vi "Tausand AB1000 Delay Sweep Example (StateMachine).vi"() -> ()   [LabVIEW 2015]
doc: "Example of a delay sweep with a Tausand Abacus AB1002 or AB1004 device.\n\nVerifies if the selected port is valid, then changes the delay in the given range. Measures a single time at each delay. Produces live graphics.\nUses only inputs in channels A and B.\nBlock diagram coded as a state machine."
uses:
  <instrlib>/Tausand AB1000/Public/Controls/counters2ch.ctl
  <instrlib>/Tausand AB1000/Examples/sub vi/delaySweep_states.ctl
  <instrlib>/Tausand AB1000/Public/Controls/deviceTypeRing.ctl
  <instrlib>/Tausand AB1000/Public/Controls/channelRing.ctl
  <instrlib>/Tausand AB1000/Tausand AB1000.lvlib
panel:
  out "counters":T1
  out "device type":T2 items=["any"=0, "AB1002"=1002, "AB1004"=1004]
  in  "step":i32=5 min=5 max=100 step=5
  out "progressStr":string
  out "current delay":i32
  out "valid data?":bool
  out "dataID":u32
  out "Total progress":dbl(slide) scale=0.0..100.0
  out "number of delays":i32
  out "delay index":i32
  out "state":T3
  out "counters array":T1[](array[typedef])
  out "wait done?":bool
  out "nextRead":u32 caption="next read in (s)"
  out "current time":timestamp
  out "wait until":timestamp
  in  "stop":bool
  out "delay array":i32[](array[numeric])
  out "BGrph":cluster{i32[], u32[]}(graph)
  out "AGrph":cluster{i32[], u32[]}(graph)
  out "coincGrph":cluster{i32[], u32[]}(graph)
  out "Delay A (ns)":u32
  out "Delay B (ns)":u32=5
  in  "Delay range (ns)":cluster{i32, i32}(slide)={-20, 20} scale=-100.0..100.0
  in  "Device settings":T4={"Sampling time (ms)"=1000, "Coincidence window (ns)"=5, "Delay A (ns)"=0, "Delay B (ns)"=0, "Sleep time A (ns)"=0, "Sleep time B (ns)"=0} {"Sleep time B (ns)" max=100 step=5; "Sleep time A (ns)" max=100 step=5; "Coincidence window (ns)" max=50000 step=5; "Sampling time (ms)" items=["1000s"=1000000, "500s"=500000, "200s"=200000, "100s"=100000, "50s"=50000, "20s"=20000, "10s"=10000, "5s"=5000, "2s"=2000, "1s"=1000, "500ms"=500, "200ms"=200, "100ms"=100, "50ms"=50, "20ms"=20, "10ms"=10, "5ms"=5, "2ms"=2, "1ms"=1]}
  out "valid device?":bool
  in  "VISA port":refnum<visa-resource-name>
  # "Overview: example doing a delay sweep in a Tausand Abacus AB1002 or AB1004 device.\nInstructions:\n1. Select the VISA port.\n2. Enter the desired settings.\n3. Run the VI.\n4. Click stop to abort the VI execution."
  # "April 2019"
  # "Set these values before running the VI."
  # "Counts at last delay:"
  # "Delay in progess:"
  # "ns"
  # "Positive delay:   A delayed,        B not delayed\nNegative delay: A not delayed, B delayed"
  # "from"
  # "to"
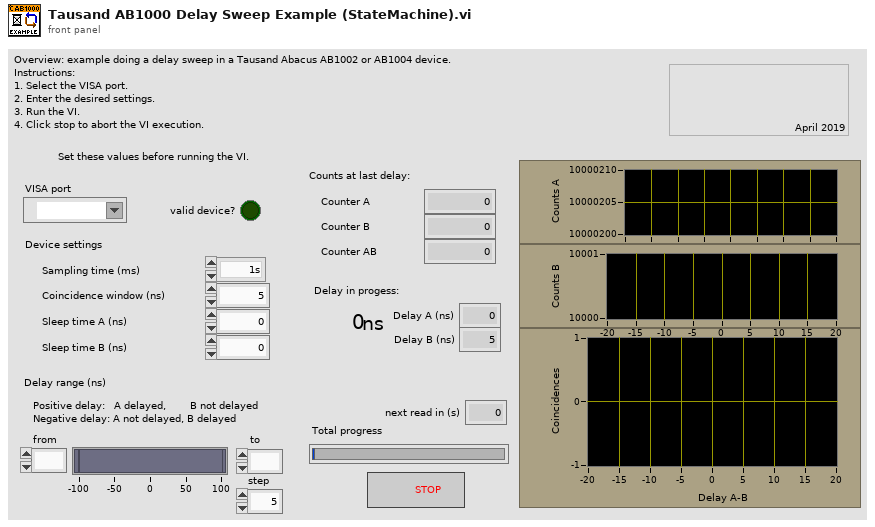
[diagram p1: front panel]
types:
  T1 = typedef "Tausand AB1000.lvlib/counters2ch.ctl" = cluster{"counter_A":u32, "counter_B":u32, "counter_AB":u32, "counters_ID":u32, "time_left":u32}
  T2 = typedef "Tausand AB1000.lvlib/deviceTypeRing.ctl" = u16
  T3 = typedef "delaySweep_states.ctl" = enum16{"update delay range", "create delay array", "verify port", "invalid port message", "create counter array", "initialize device", "set delay", "set wait timer", "wait sampling time", "read data", "graph data", "increase index", "repeat measurement", "close device", "end state"}
  T4 = cluster{"Sampling time (ms)":u32, "Coincidence window (ns)":u32, "Delay A (ns)":u32, "Delay B (ns)":u32, "Sleep time A (ns)":u32, "Sleep time B (ns)":u32}
  T5 = typedef "Tausand AB1000.lvlib/channelRing.ctl" = u8
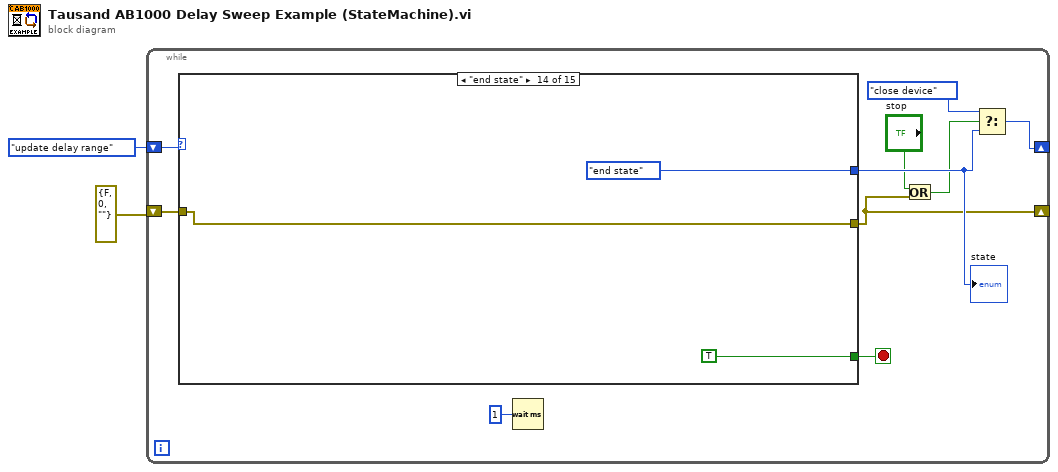
[diagram p0: block diagram]
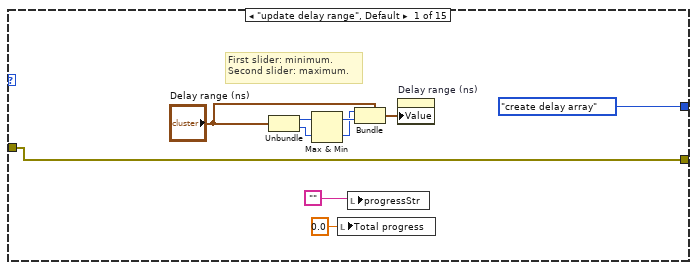
[diagram p2: hidden frame]
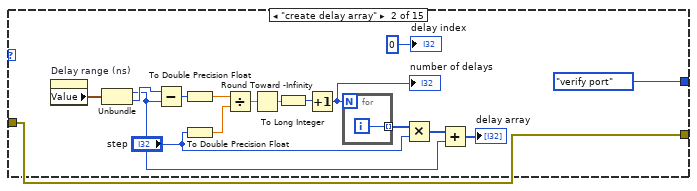
[diagram p3: hidden frame]
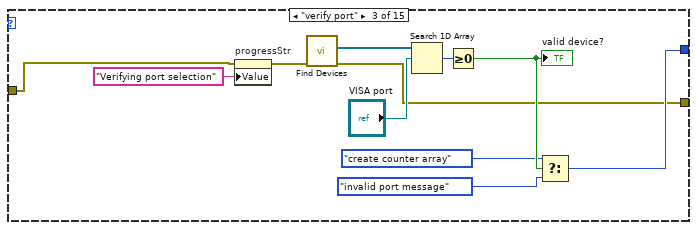
[diagram p4: hidden frame]
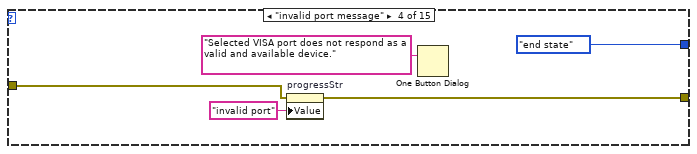
[diagram p5: hidden frame]
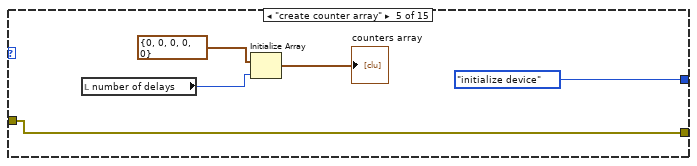
[diagram p6: hidden frame]
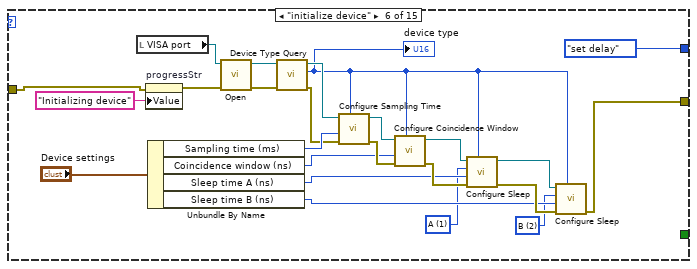
[diagram p7: hidden frame]
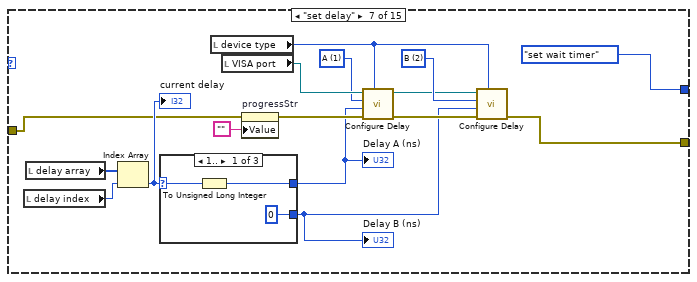
[diagram p8: hidden frame]
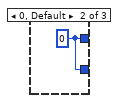
[diagram p9: hidden frame]
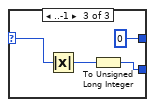
[diagram p10: hidden frame]
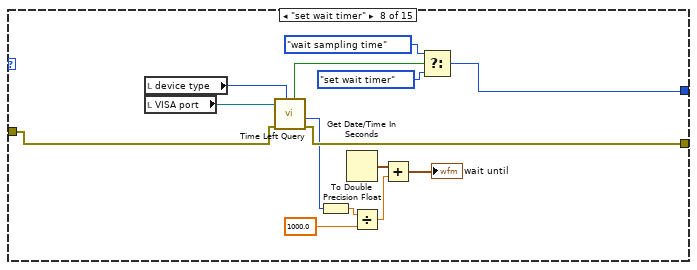
[diagram p11: hidden frame]
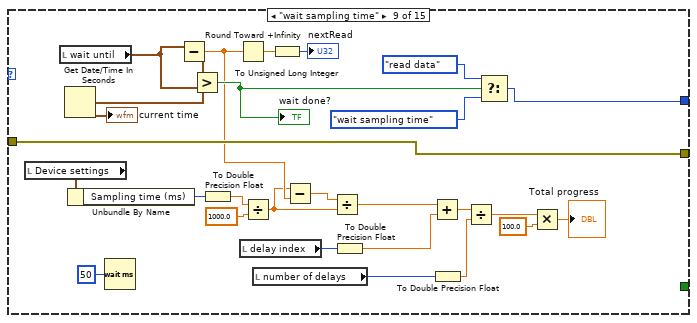
[diagram p12: hidden frame]
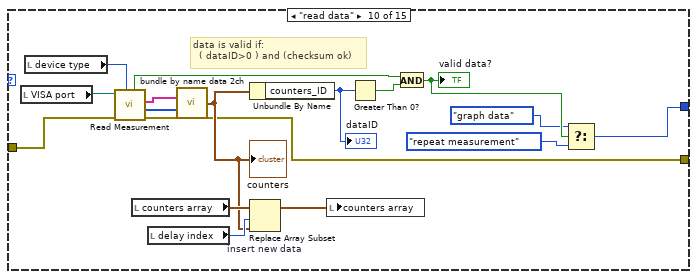
[diagram p13: hidden frame]
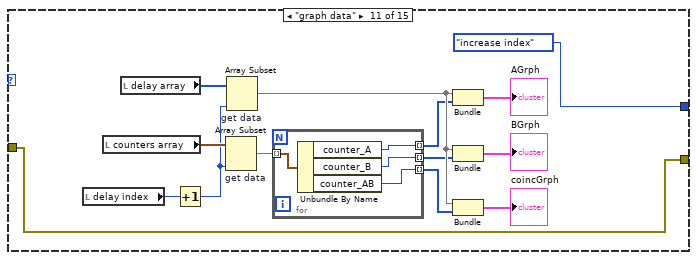
[diagram p14: hidden frame]
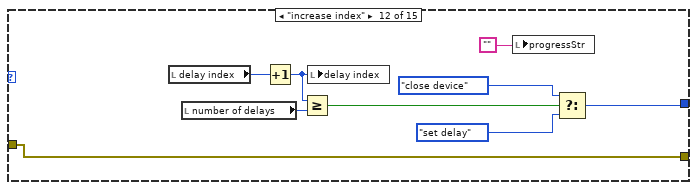
[diagram p15: hidden frame]
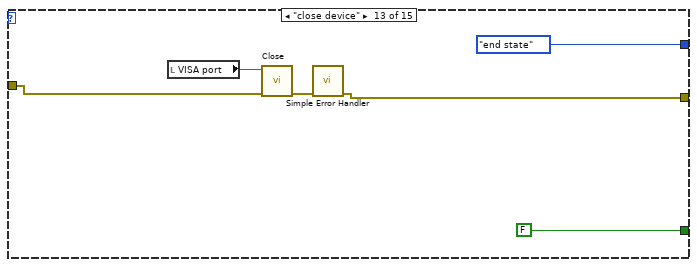
[diagram p16: hidden frame]
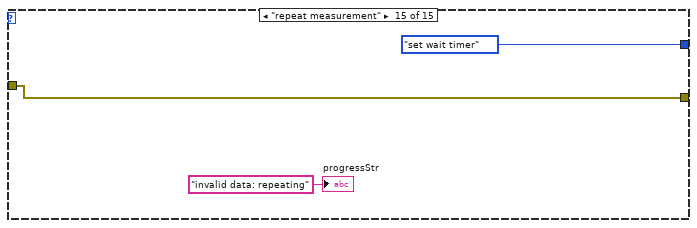
[diagram p17: hidden frame]
diagram:
  n1 = while {
    shift-right: [w6] -> _
    shift-left: delaySweep_states."update delay range" -> [w12]
    shift-right: [w5] -> _
    shift-left: errorcluster {"status"=FALSE, "code"=0, "source"=""} ("error in (no error)") -> [w10]
    stop <- w9 stop-if-true
    n2 = case shown="\"end state\"" w12 {
      tunnel: [delaySweep_states."create delay array" delaySweep_states."verify port" w46 delaySweep_states."end state" delaySweep_states."initialize device" delaySweep_states."set delay" delaySweep_states."set wait timer" w112 w141 w159 delaySweep_states."increase index" w186 delaySweep_states."end state" delaySweep_states."end state" delaySweep_states."set wait timer"] -> w7
      tunnel: [_ _ _ _ _ _ _ _ _ _ _ _ FALSE TRUE _] -> w9
      tunnel: w10 -> [w15 w28 w43 w53 w58 w82 w96 w117 w149 w156 w179 w193 w196 w200 w205]
      tunnel: [w15 w28 w41 w52 w58 w65 w87 w116 w149 w151 w179 w193 w195 w200 w205] -> w5
      frame "update delay range", Default {
        # "First slider: minimum.\nSecond slider: maximum."
        n3 = Unbundle("Delay range (ns)") -> (w22:i32, w17:i32)
        n4 = Max & Min(x=w22, y=w17) -> (max(x,y)=w19:i32, min(x,y)=w16:i32)
        n5 = local write "Total progress"(0.0 ("Total progress")) -> ()
        n6 = local write "progressStr"("") -> ()
        n7 = Bundle(cluster="Delay range (ns)", w16, w19) -> (w20:cluster{i32, i32})
        n8 = property on="Delay range (ns)" class="Slide (strict)"("Value"=w20) -> ()  [unwired: 2 in, 2 out]
      }
      frame "create delay array" {
        n9 = property on="Delay range (ns)" class="Slide (strict)"() -> ("Value"=w31:cluster{i32, i32})  [unwired: 2 in, 2 out]
        n10 = Unbundle(w31) -> (w29:i32, w30:i32)
        n11 = Subtract(x=w30, y=w29) -> (x-y=w38:i32)
        n12 = To Double Precision Float(number=w38) -> (double precision float=w36:dbl)
        n13 = To Double Precision Float(number="step") -> (double precision float=w35:dbl)
        n14 = Divide(x=w36, y=w35) -> (x/y=w24:dbl)
        n15 = Round Toward -Infinity(1:w24) -> (0:w23:dbl)
        n16 = To Long Integer(number=w23) -> (32bit integer=w32:i32)
        n17 = Increment(x=w32) -> (x+1=w25:i32)
        "number of delays" <- w25
        n18 = for {
          N: w25 -> [_]
          tunnel: [w40] -> w37 mode=indexing
          i -> [w40]
        }
        n19 = Multiply(x=w37, y="step") -> (x*y=w33:i32[])
        n20 = Add(x=w33, y=w29) -> (x+y=→"delay array":i32[])
        "delay index" <- 0 ("delay index")
      }
      frame "verify port" {
        n21 = property on="progressStr" class="Str"(error in=w43, "Value"="Verifying port selection" ("progressStr")) -> (error out=w42:errorcluster)  [unwired: 1 in, 1 out]
        n22 = call <instrlib>:"Find Devices.vi"("error in (no error)"=w42) -> ("error out"=w41:errorcluster, "Abacus VISAs"=w49:refnum<visa-resource-name>[])  [unwired: 8 in, 1 out]
        n23 = Search 1D Array(1D array=w49, element="VISA port") -> (index of element=w51:i32)  [unwired: 1 in]
        n24 = Greater Or Equal To 0?(x=w51) -> (x >= 0?=w48:bool)
        "valid device?" <- w48
        n25 = Select(t=delaySweep_states."create counter array", s=w48, f=delaySweep_states."invalid port message") -> (s? t:f=w46:T3)
      }
      frame "invalid port message" {
        n26 = property on="progressStr" class="Str"(error in=w53, "Value"="invalid port" ("progressStr")) -> (error out=w52:errorcluster)  [unwired: 1 in, 1 out]
        n27 = One Button Dialog(message="Selected VISA port does not respond as a valid and available device.") -> ()  [unwired: 1 in, 1 out]
      }
      frame "create counter array" {
        n28 = local read "number of delays"() -> (w57:i32)
        n29 = Initialize Array "Initialize Array"(T1 {"counter_A"=0, "counter_B"=0, "counter_AB"=0, "counters_ID"=0, "time_left"=0} ("counters"), w57) -> (→"counters array":T1[])
      }
      frame "initialize device" {
        w67 = T5 2 items=["none", "A", "B", "C", "D", "E", "F", "G", "H"] ("channel")
        w68 = T5 1 items=["none", "A", "B", "C", "D", "E", "F", "G", "H"] ("channel")
        n30 = local read "VISA port"() -> (w84:refnum<visa-resource-name>)
        n31 = property on="progressStr" class="Str"(error in=w82, "Value"="Initializing device" ("progressStr")) -> (error out=w81:errorcluster)  [unwired: 1 in, 1 out]
        n32 = Unbundle By Name("Device settings") -> ("Sampling time (ms)"=w72:u32, "Coincidence window (ns)"=w71:u32, "Sleep time A (ns)"=w70:u32, "Sleep time B (ns)"=w69:u32)
        n33 = call <instrlib>:"Open.vi"("error in (no error)"=w81, "VISA resource name"=w84) -> ("error out"=w79:errorcluster, "VISA resource name out"=w80:refnum<visa-resource-name>)  [unwired: 8 in]
        n34 = call <instrlib>:"Device Type Query.vi"("error in (no error)"=w79, "VISA Refnum in"=w80) -> ("error out"=w66:errorcluster, "device type"=w62:T2, "VISA Refnum out"=w64:refnum<visa-resource-name>)  [unwired: 7 in]
        "device type" <- w62
        n35 = call <instrlib>:"Configure Sampling Time.vi"("device type"=w62, "error in (no error)"=w66, "value (1000 ms)"=w72, "VISA Refnum in"=w64) -> ("error out"=w78:errorcluster, "VISA Refnum out"=w77:refnum<visa-resource-name>)  [unwired: 5 in, 1 out]
        n36 = call <instrlib>:"Configure Coincidence Window.vi"("device type"=w62, "error in (no error)"=w78, "value ns (10ns)"=w71, "VISA Refnum in"=w77) -> ("error out"=w75:errorcluster, "VISA Refnum out"=w76:refnum<visa-resource-name>)  [unwired: 5 in, 1 out]
        n37 = call <instrlib>:"Configure Sleep.vi"("device type"=w62, "error in (no error)"=w75, "value (0 ns)"=w70, "channel"=w68, "VISA Refnum in"=w76) -> ("error out"=w73:errorcluster, "VISA Refnum out"=w74:refnum<visa-resource-name>)  [unwired: 4 in, 1 out]
        n38 = call <instrlib>:"Configure Sleep.vi"("device type"=w62, "error in (no error)"=w73, "value (0 ns)"=w69, "channel"=w67, "VISA Refnum in"=w74) -> ("error out"=w65:errorcluster)  [unwired: 4 in, 2 out]
      }
      frame "set delay" {
        w90 = T5 2 items=["none", "A", "B", "C", "D", "E", "F", "G", "H"] ("channel")
        w91 = T5 1 items=["none", "A", "B", "C", "D", "E", "F", "G", "H"] ("channel")
        n39 = local read "delay index"() -> (w98:i32)
        n40 = local read "delay array"() -> (w100:i32[])
        n41 = Index Array(array=w100, index=w98) -> (element=w99:i32)
        "current delay" <- w99
        n42 = case shown="1.." w99 {
          selector: w99 -> [w102 _ w107]
          tunnel: [u32 0 w105 w109] -> w89
          tunnel: [w104 w105 u32 0 ("Delay A (ns)")] -> w92
          frame 1.. {
            n43 = To Unsigned Long Integer(number=w102) -> (unsigned 32bit integer=w104:u32)
          }
          frame 0, Default {
            w105 = u32 0 ("Delay A (ns)")
          }
          frame ..-1 {
            n44 = Absolute Value(x=w107) -> (abs(x)=w106:i32)
            n45 = To Unsigned Long Integer(number=w106) -> (unsigned 32bit integer=w109:u32)
          }
        }
        "Delay A (ns)" <- w92
        "Delay B (ns)" <- w89
        n46 = local read "device type"() -> (w86:T2)
        n47 = local read "VISA port"() -> (w95:refnum<visa-resource-name>)
        n48 = property on="progressStr" class="Str"(error in=w96, "Value"="" ("progressStr")) -> (error out=w93:errorcluster)  [unwired: 1 in, 1 out]
        n49 = call <instrlib>:"Configure Delay.vi"("device type"=w86, "error in (no error)"=w93, "value (0 ns)"=w92, "channel"=w91, "VISA Refnum in"=w95) -> ("error out"=w94:errorcluster, "VISA Refnum out"=w88:refnum<visa-resource-name>)  [unwired: 4 in, 1 out]
        n50 = call <instrlib>:"Configure Delay.vi"("device type"=w86, "error in (no error)"=w94, "value (0 ns)"=w89, "channel"=w90, "VISA Refnum in"=w88) -> ("error out"=w87:errorcluster)  [unwired: 4 in, 2 out]
      }
      frame "set wait timer" {
        n51 = local read "device type"() -> (w110:T2)
        n52 = local read "VISA port"() -> (w118:refnum<visa-resource-name>)
        n53 = call <instrlib>:"Time Left Query.vi"("device type"=w110, "error in (no error)"=w117, "VISA Refnum in"=w118) -> ("error out"=w116:errorcluster, "time left ms out"=w115:u32, "checksum ok?"=w114:bool)  [unwired: 5 in, 1 out]
        n54 = To Double Precision Float(number=w115) -> (double precision float=w119:dbl)
        n55 = Get Date/Time In Seconds() -> (seconds since 1Jan1904=w122:timestamp)
        n56 = Divide(x=w119, y=1000.0) -> (x/y=w120:dbl)
        n57 = Add(x=w122, y=w120) -> (x+y=→"wait until":timestamp)
        n58 = Select(t=delaySweep_states."wait sampling time", s=w114, f=delaySweep_states."set wait timer") -> (s? t:f=w112:T3)
      }
      frame "wait sampling time" {
        n59 = local read "Device settings"() -> (w128:T4)
        n60 = local read "wait until"() -> (w147:timestamp)
        n61 = Get Date/Time In Seconds() -> (seconds since 1Jan1904=w148:timestamp)
        "current time" <- w148
        n62 = Unbundle By Name(w128) -> ("Sampling time (ms)"=w125:u32)
        n63 = Wait (ms)(milliseconds to wait=u32 50) -> ()  [unwired: 1 out]
        n64 = Subtract(x=w147, y=w148) -> (x-y=w136:dbl)
        n65 = Greater?(x=w148, y=w147) -> (0:w144:bool)
        "wait done?" <- w144
        n66 = To Double Precision Float(number=w125) -> (double precision float=w127:dbl)
        n67 = Round Toward +Infinity(x=w136) -> (ceil(x): smallest int >= x=w146:dbl)
        n68 = local read "delay index"() -> (w132:i32)
        n69 = Divide(x=w127, y=1000.0) -> (x/y=w124:dbl)
        n70 = local read "number of delays"() -> (w133:i32)
        n71 = To Unsigned Long Integer(number=w146) -> (unsigned 32bit integer=→"nextRead":u32)
        n72 = Subtract(x=w124, y=w136) -> (x-y=w135:dbl)
        n73 = Divide(x=w135, y=w124) -> (x/y=w134:dbl)
        n74 = To Double Precision Float(number=w132) -> (double precision float=w131:dbl)
        n75 = Add(x=w134, y=w131) -> (x+y=w137:dbl)
        n76 = To Double Precision Float(number=w133) -> (double precision float=w129:dbl)
        n77 = Divide(x=w137, y=w129) -> (x/y=w139:dbl)
        n78 = Select(t=delaySweep_states."read data", s=w144, f=delaySweep_states."wait sampling time") -> (s? t:f=w141:T3)
        n79 = Multiply(x=w139, y=100.0) -> (x*y=→"Total progress":dbl)
      }
      frame "read data" {
        # "data is valid if:\n  ( dataID>0 ) and (checksum ok)"
        n80 = local read "VISA port"() -> (w157:refnum<visa-resource-name>)
        n81 = local read "device type"() -> (w150:T2)
        n82 = call <instrlib>:"Read Measurement.vi"("device type"=w150, "error in (no error)"=w156, "VISA Refnum in"=w157) -> ("error out"=w151:errorcluster, "values"=w154:u32[], "labels"=w155:string[], "checksum ok?"=w152:bool)  [unwired: 3 in, 2 out]
        n83 = local read "counters array"() -> (w165:T1[])
        n84 = local read "delay index"() -> (w164:i32)
        n85 = call <instrlib>:"bundle by name data 2ch.vi"("names"=w155, "values"=w154) -> ("output cluster 2ch"=w153:T1)  [unwired: 13 in]
        "counters" <- w153
        n86 = Unbundle By Name(w153) -> ("counters_ID"=w158:u32)
        "dataID" <- w158
        n87 = Replace Array Subset "insert new data"(array=w165, new element=w153, index=w164) -> (w166:T1[])
        n88 = local write "counters array"(w166) -> ()
        n89 = Greater Than 0?(x=w158) -> (x > 0?=w163:bool)
        n90 = And(x=w152, y=w163) -> (x .and. y?=w162:bool)
        "valid data?" <- w162
        n91 = Select(t=delaySweep_states."graph data", s=w162, f=delaySweep_states."repeat measurement") -> (s? t:f=w159:T3)
      }
      frame "graph data" {
        n92 = local read "delay index"() -> (w168:i32)
        n93 = local read "counters array"() -> (w169:T1[])
        n94 = local read "delay array"() -> (w170:i32[])
        n95 = Increment(x=w168) -> (x+1=w167:i32)
        n96 = Array Subset "get data"(array=w169, length=w167) -> (w174:T1[])  [unwired: 1 in]
        n97 = Array Subset "get data"(array=w170, length=w167) -> (w175:i32[])  [unwired: 1 in]
        n98 = for {
          tunnel: w174 -> [w184] mode=indexing
          tunnel: [w183] -> w173 mode=indexing
          tunnel: [w182] -> w172 mode=indexing
          tunnel: [w181] -> w171 mode=indexing
          n99 = Unbundle By Name(w184) -> ("counter_A"=w183:u32, "counter_B"=w182:u32, "counter_AB"=w181:u32)
        }
        n100 = Bundle(w175, w173) -> (→"AGrph":cluster{i32[], u32[]})  [unwired: 1 in]
        n101 = Bundle(w175, w172) -> (→"BGrph":cluster{i32[], u32[]})  [unwired: 1 in]
        n102 = Bundle(w175, w171) -> (→"coincGrph":cluster{i32[], u32[]})  [unwired: 1 in]
      }
      frame "increase index" {
        n103 = local read "delay index"() -> (w192:i32)
        n104 = local read "number of delays"() -> (w190:i32)
        n105 = Increment(x=w192) -> (x+1=w191:i32)
        n106 = Greater Or Equal?(x=w191, y=w190) -> (x >= y?=w189:bool)
        n107 = local write "delay index"(w191) -> ()
        n108 = local write "progressStr"("") -> ()
        n109 = Select(t=delaySweep_states."close device", s=w189, f=delaySweep_states."set delay") -> (s? t:f=w186:T3)
      }
      frame "close device" {
        n110 = local read "VISA port"() -> (w194:refnum<visa-resource-name>)
        n111 = call <instrlib>:"Close.vi"("error in (no error)"=w196, "VISA resource name"=w194) -> ("error out"=w197:errorcluster)  [unwired: 9 in]
        n112 = call <vilib>:"Simple Error Handler.vi"("error in (no error)"=w197) -> ("error out"=w195:errorcluster)  [unwired: 4 in, 4 out]
      }
      frame "end state" {
      }
      frame "repeat measurement" {
        "progressStr" <- "invalid data: repeating" ("repeatingStr")
      }
    }
    "state" <- w7
    n113 = Wait (ms)(milliseconds to wait=u32 1) -> ()  [unwired: 1 out]
    n114 = Or(x="stop", y=w5) -> (x .or. y?=w3:bool)
    n115 = Select(t=delaySweep_states."close device", s=w3, f=w7) -> (s? t:f=w6:T3)
  }
